vi "ENPH354_A4Q4.vi"() -> ()   [LabVIEW 2020]
uses:
  <vilib>/Utility/file.llb/Read Delimited Spreadsheet (DBL).vi
panel:
  out "Average Photon Energy [eV]":dbl
  out "Counts vs Photon Energy":cluster{"X":dbl[], "Y":dbl[]}[](graph)
  in  "Corrected WLED Emission":path
  # "ENPH354 Assignment 4 Q4"
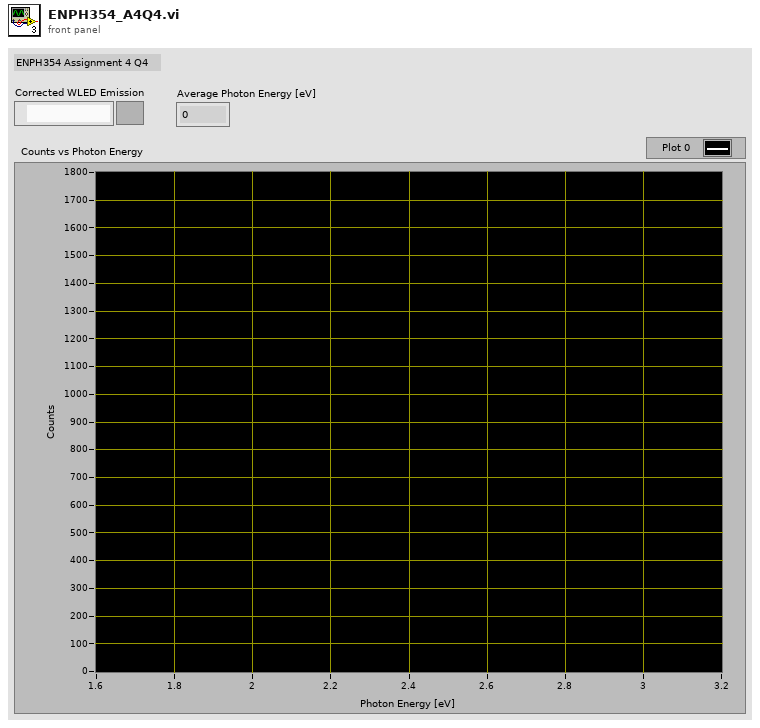
[diagram p1: front panel]
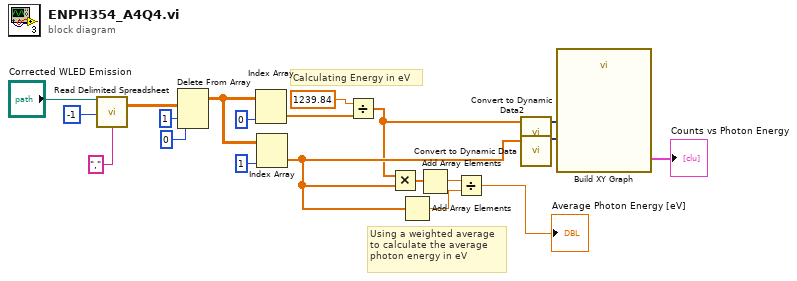
[diagram p0: block diagram]
diagram:
  # "Using a weighted average\nto calculate the average \nphoton energy in eV"
  # "Calculating Energy in eV"
  n1 = call-poly <vilib>:"Read Delimited Spreadsheet.vi"("file path (dialog if empty)"="Corrected WLED Emission", "number of rows (all:-1)"=-1, "delimiter (\\t)"="," ("delimiter (\\t)")) -> ("all rows"=w17:dbl[][])  [unwired: 7 in, 5 out]
  n2 = Delete From Array(array=w17, length=1, index (row)=0) -> (array with subset deleted=w12:dbl[][])  [unwired: 1 in, 1 out]
  n3 = Index Array(array=w12, index (col)=0) -> (element=w3:dbl[])  [unwired: 1 in]
  n4 = Index Array(array=w12, index (col)=1) -> (element=w2:dbl[])  [unwired: 1 in]
  n5 = Divide(x=1239.84, y=w3) -> (x/y=w1:dbl[])
  n6 = Multiply(x=w1, y=w2) -> (x*y=w7:dbl[])
  n7 = Add Array Elements(numeric array=w2) -> (sum=w4:dbl)
  n8 = Add Array Elements(numeric array=w7) -> (sum=w6:dbl)
  n9 = Divide(x=w6, y=w4) -> (x/y=→"Average Photon Energy [eV]":dbl)
  n10 = call "Convert to Dynamic Data2"("Array"=w1) -> ("Dynamic Data Type"=w8:dynamicdata)  [unwired: 3 in]
  n11 = call "Convert to Dynamic Data"("Array"=w2) -> ("Dynamic Data Type"=w10:dynamicdata)  [unwired: 3 in]
  n12 = call "Build XY Graph"("Y Input"=w10, "X Input"=w8) -> ("XY Graph"=→"Counts vs Photon Energy":cluster{"X":dbl[], "Y":dbl[]}[])  [unwired: 8 in, 1 out]
